vi "sub_2D Array to 1D.vi"(1 "2D Array":fxp<+/-,32,16>[][](array[numeric])) -> (0 "Random 1D Array":fxp<+/-,32,16>[](array[numeric]) format="%.21g")   [LabVIEW 2015]
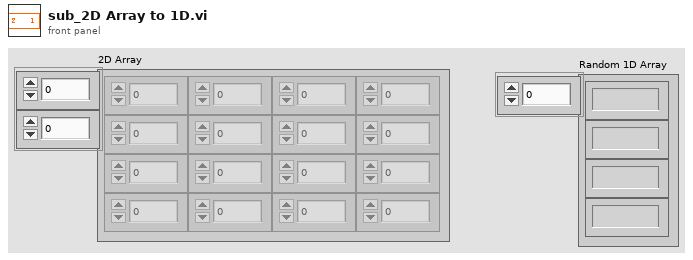
[diagram p1: front panel]
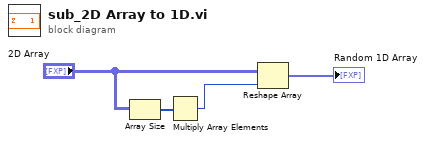
[diagram p0: block diagram]
diagram:
  n1 = Array Size(array="2D Array") -> (size(s)=w3:i32[])
  n2 = Multiply Array Elements(1:w3) -> (0:w2:i32)
  n3 = Reshape Array("2D Array", w2) -> (→"Random 1D Array":fxp<+/-,32,16>[])
